vi "Duplicate Name Error Test.vi"() -> (0 "error out":errorcluster, 1 "Success Error on Replace Line":bool, 2 "Success Error on Write Lines":bool, 3 "Success Error on Add":bool)   [LabVIEW 2015, in "PID Module 2 tests.lvlib"]
doc: "Tests the Add Line and Remove Line functions."
uses:
  PID Module 2 tests.lvlib
  module/configuration/Get Line Name.vi
  <vilib>/NI/Tag Bus Module Framework/module configuration/FindDuplicate.vi
  <vilib>/Utility/error.llb/Error Cluster From Error Code.vi
  module/configuration/PID Module 2 configuration.lvclass
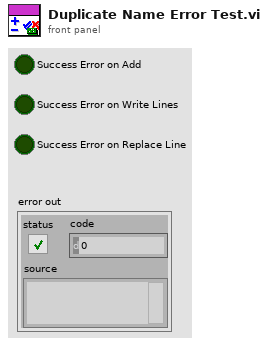
[diagram p1: front panel]
types:
  T1 = typedef "PID Module 2 configuration.lvclass/Line.ctl" = cluster{"PID ID":string, "Setpoint":refnum<class "TBM channel.lvclass">, "Variable":refnum<class "TBM channel.lvclass">, "Output":refnum<class "TBM channel.lvclass">, "Output High":refnum<class "TBM channel.lvclass">, "Output Low":refnum<class "TBM channel.lvclass">, "P":refnum<class "TBM channel.lvclass">, "I":refnum<class "TBM channel.lvclass">, "D":refnum<class "TBM channel.lvclass">}
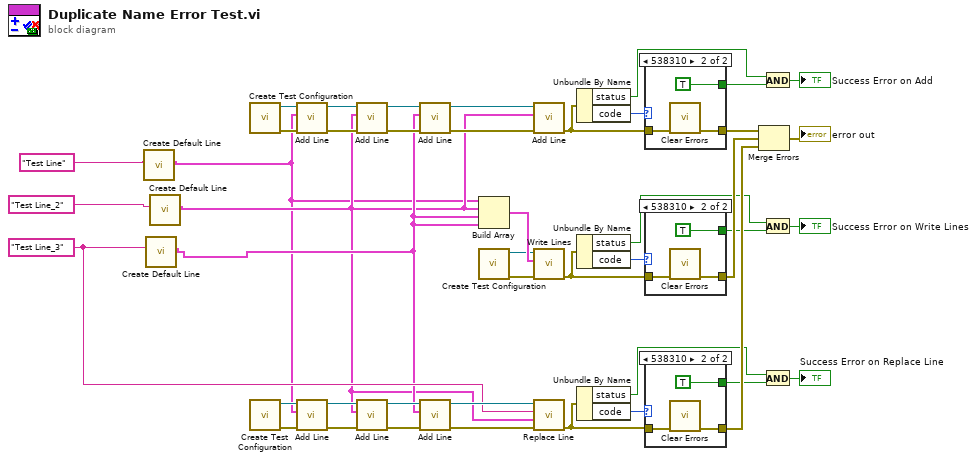
[diagram p0: block diagram]
diagram:
  w6 = "Test Line_3" ("channel name")
  n1 = call "Create Default Line.vi"("Line Name"="Test Line" ("channel name")) -> ("Default Line"=w1:T1)  [unwired: 10 in]
  n2 = call "Create Default Line.vi"("Line Name"=w6) -> ("Default Line"=w5:T1)  [unwired: 10 in]
  n3 = call "Create Default Line.vi"("Line Name"="Test Line_2" ("channel name")) -> ("Default Line"=w4:T1)  [unwired: 10 in]
  n4 = call "Create Test Configuration.vi"() -> ("error out"=w43:errorcluster, "Module Configuration"=w44:refnum<class "PID Module 2 configuration.lvclass">)  [unwired: 6 in, 4 out]
  n5 = call "Create Test Configuration.vi"() -> ("error out"=w23:errorcluster, "Module Configuration"=w22:refnum<class "PID Module 2 configuration.lvclass">)  [unwired: 6 in, 4 out]
  n6 = call "Add Line.vi"("error in"=w43, "Line"=w1, "PID Module 2 configuration in"=w44) -> ("error out"=w42:errorcluster, "PID Module 2 configuration out"=w39:refnum<class "PID Module 2 configuration.lvclass">)  [unwired: 6 in, 1 out]
  n7 = call "Add Line.vi"("error in"=w23, "Line"=w1, "PID Module 2 configuration in"=w22) -> ("error out"=w24:errorcluster, "PID Module 2 configuration out"=w27:refnum<class "PID Module 2 configuration.lvclass">)  [unwired: 6 in, 1 out]
  n8 = call "Add Line.vi"("error in"=w42, "Line"=w4, "PID Module 2 configuration in"=w39) -> ("error out"=w41:errorcluster, "PID Module 2 configuration out"=w40:refnum<class "PID Module 2 configuration.lvclass">)  [unwired: 6 in, 1 out]
  n9 = call "Add Line.vi"("error in"=w24, "Line"=w4, "PID Module 2 configuration in"=w27) -> ("error out"=w25:errorcluster, "PID Module 2 configuration out"=w26:refnum<class "PID Module 2 configuration.lvclass">)  [unwired: 6 in, 1 out]
  n10 = call "Add Line.vi"("error in"=w41, "Line"=w5, "PID Module 2 configuration in"=w40) -> ("error out"=w37:errorcluster, "PID Module 2 configuration out"=w38:refnum<class "PID Module 2 configuration.lvclass">)  [unwired: 6 in, 1 out]
  n11 = call "Add Line.vi"("error in"=w25, "Line"=w5, "PID Module 2 configuration in"=w26) -> ("error out"=w20:errorcluster, "PID Module 2 configuration out"=w21:refnum<class "PID Module 2 configuration.lvclass">)  [unwired: 6 in, 1 out]
  n12 = Build Array(w1, w4, w5, w5) -> (w34:T1[])
  n13 = call "Create Test Configuration.vi"() -> ("error out"=w19:errorcluster, "Module Configuration"=w33:refnum<class "PID Module 2 configuration.lvclass">)  [unwired: 6 in, 4 out]
  n14 = call "Add Line.vi"("error in"=w37, "Line"=w4, "PID Module 2 configuration in"=w38) -> ("error out"=w35:errorcluster)  [unwired: 6 in, 2 out]
  n15 = call "Write Lines.vi"("error in (no error)"=w19, "Lines"=w34, "PID Module 2 configuration in"=w33) -> ("error out"=w31:errorcluster)  [unwired: 7 in, 1 out]
  n16 = call "Replace Line.vi"("error in"=w20, "New Line"=w4, "Line Name"=w6, "PID Module 2 configuration in"=w21) -> ("error out"=w17:errorcluster)  [unwired: 5 in, 2 out]
  n17 = Unbundle By Name(w35) -> ("status"=w14:bool, "code"=w36:i32)
  n18 = Unbundle By Name(w31) -> ("status"=w9:bool, "code"=w32:i32)
  n19 = Unbundle By Name(w17) -> ("status"=w10:bool, "code"=w18:i32)
  n20 = case shown="538310" w36 {
    tunnel: w35 -> [w45 w48]
    tunnel: [w45 w47] -> w30
    tunnel: [_ TRUE ("Success Error on Add")] -> w15
    frame 0, Default {
    }
    frame 538310 {
      n21 = call <vilib>:"Clear Errors.vi"("error in (no error)"=w48) -> ("error out"=w47:errorcluster)  [unwired: 5 in, 1 out]
    }
  }
  n22 = case shown="538310" w32 {
    tunnel: w31 -> [w49 w52]
    tunnel: [w49 w51] -> w29
    tunnel: [_ TRUE ("Success Error on Add")] -> w8
    frame 0, Default {
    }
    frame 538310 {
      n23 = call <vilib>:"Clear Errors.vi"("error in (no error)"=w52) -> ("error out"=w51:errorcluster)  [unwired: 5 in, 1 out]
    }
  }
  n24 = case shown="538310" w18 {
    tunnel: w17 -> [w53 w56]
    tunnel: [w53 w55] -> w16
    tunnel: [_ TRUE ("Success Error on Add")] -> w11
    frame 0, Default {
    }
    frame 538310 {
      n25 = call <vilib>:"Clear Errors.vi"("error in (no error)"=w56) -> ("error out"=w55:errorcluster)  [unwired: 5 in, 1 out]
    }
  }
  n26 = Merge Errors(w30, w29, w16) -> (→"error out":errorcluster)
  n27 = And(x=w14, y=w15) -> (x .and. y?=→"Success Error on Add":bool)
  n28 = And(x=w9, y=w8) -> (x .and. y?=→"Success Error on Write Lines":bool)
  n29 = And(x=w10, y=w11) -> (x .and. y?=→"Success Error on Replace Line":bool)
